vi "Test Copy from Pixmap.vi"(8 "error in (no error)":errorcluster, 11 "Test Case In":refnum<class "Image.lvclass">) -> (0 "error out":errorcluster, 3 "Test Case Out":refnum<class "Image.lvclass">)   [LabVIEW 2020, in "g_ar_toolkit.test.lvlib" / "Image.lvclass"]
uses:
  Image.lvclass
  C:/Program Files (x86)/National Instruments/LabVIEW 2020/vi.lib/Astemes/LUnit/Test Case.lvclass
  <vilib>/Astemes/LUnit/Test Case.lvclass/Test Case.ctl
  g_ar_toolkit.image/CreateEmptyImageARGB.vi
  g_ar_toolkit.image/CopyPixmapToImageIgnoreMaskARGB.vi
  4993e8ee-a06a-463a-9684-69129f64d5ce.vi
  g_ar_toolkit.image/CreateEmptyImageARGB.vi/3321fa97-f432-4e1e-8db9-a0df79aed21b.vi
  g_ar_toolkit.image/CopyPixmapToImageIgnoreMaskARGB.vi/80b1166a-8c06-443b-b271-eb6a715622f7.vi
  <vilib>/Astemes/LUnit/Append Pass Result.vi
  <vilib>/Astemes/LUnit/Append Fail Result.vi
  <vilib>/Astemes/LUnit/Describe Comparison.vi
  <vilib>/Astemes/LUnit/Compare Variants.vi
  g_ar_toolkit.image/FixPixmapColourArraySize.vi
  <vilib>/Astemes/LUnit/Variant to string.vi
  g_ar_toolkit.image/Default8bitColourMap.vi
  <vilib>/Utility/Data Type/Get Type Information.vi
  <vilib>/Utility/LVClass/Get LV Class Name.vi
  g_ar_toolkit.image/ARGBColourToU32.vi
  <vilib>/Utility/error.llb/Error Cluster From Error Code.vi
  Image.lvclass/Image.ctl
  g_ar_toolkit.image/g_ar_toolkit.image.lvlib
panel:
  out "output cluster":T1(array[cluster]) {"data value" format="%.0x"; "24-bit pixmap" format="%.0x"}
  out "Array":picture[](array[picture])
  out "data value":u32[][][](array[numeric]) format="%.0x"
  out "Picture":picture
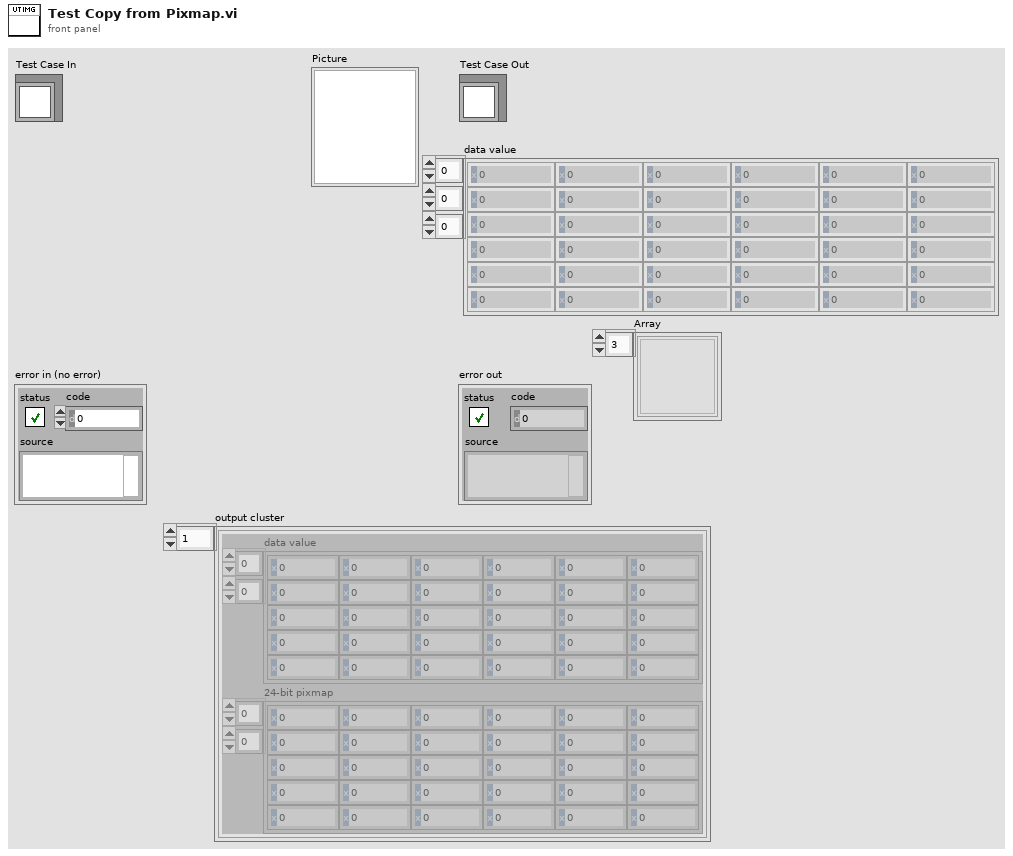
[diagram p1: front panel]
types:
  T1 = cluster{"data value":u32[][], "24-bit pixmap":u32[][]}[]
  T2 = cluster{"left":i16, "top":i16, "right":i16, "bottom":i16}
  T3 = typedef "imagedata.ctl" = cluster{"image type":i32, "image depth":i32, "image":u8[], "mask":u8[], "colors":u32[], "Rectangle":cluster{"left":i16, "top":i16, "right":i16, "bottom":i16}}
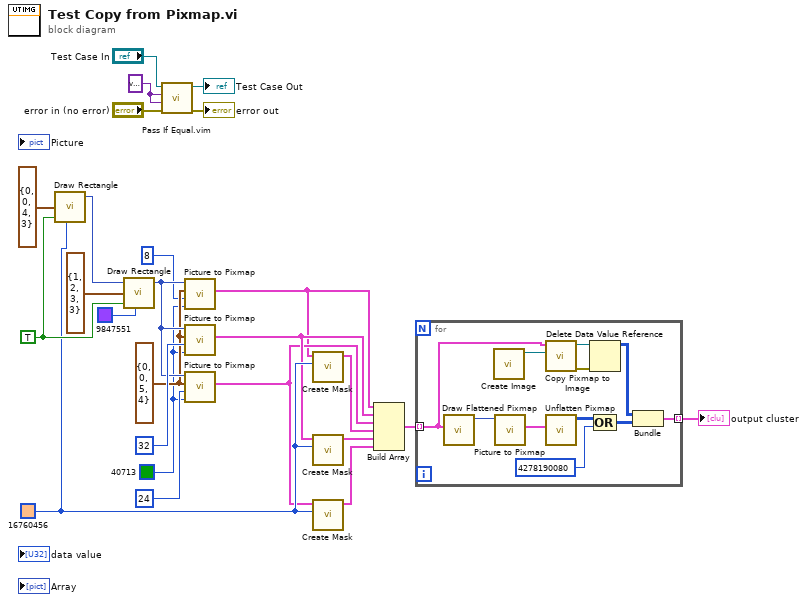
[diagram p0: block diagram]
diagram:
  w15 = TRUE ("fill?(F)")
  w16 = variant ("Expected")
  w12 = T2 {"left"=0, "top"=0, "right"=5, "bottom"=4} ("rect")
  w10 = u32 40713 ("Background Color")
  w9 = u32 16760456 ("color(black)")
  n1 = call <vilib>:"Draw Rectangle.vi"("rect"=T2 {"left"=0, "top"=0, "right"=4, "bottom"=3}, "fill?(F)"=w15, "color(black)"=w9) -> ("new picture"=w21:picture)  [unwired: 6 in]
  n2 = call <vilib>:"Draw Rectangle.vi"("picture"=w21, "rect"=T2 {"left"=1, "top"=2, "right"=3, "bottom"=3}, "fill?(F)"=w15, "color(black)"=u32 9847551) -> ("new picture"=w13:picture)  [unwired: 5 in]
  n3 = call "Pass If Equal.vim"("error in (no error)"="error in (no error)", "Actual"=w16, "Expected"=w16, "LUnit Test Case In"="Test Case In") -> ("error out"=→"error out":errorcluster, "LUnit Test Case Out"=→"Test Case Out":refnum<class "Image.lvclass">)  [unwired: 6 in]
  n4 = call <vilib>:"Picture to Pixmap.vi"("Background Color"=w10, "depth"=8, "rect"=w12, "picture"=w13) -> ("image data"=w1:T3)  [unwired: 6 in, 1 out]
  n5 = call <vilib>:"Picture to Pixmap.vi"("Background Color"=w10, "depth"=32, "rect"=w12, "picture"=w13) -> ("image data"=w8:T3)  [unwired: 6 in, 1 out]
  n6 = call <vilib>:"Picture to Pixmap.vi"("Background Color"=w10, "depth"=24, "rect"=w12, "picture"=w13) -> ("image data"=w2:T3)  [unwired: 6 in, 1 out]
  n7 = call <vilib>:"Create Mask.vi"("Mask Color (Black)"=w9, "image data"=w1) -> ("image data"=w7:T3)  [unwired: 9 in]
  n8 = call <vilib>:"Create Mask.vi"("Mask Color (Black)"=w9, "image data"=w8) -> ("image data"=w6:T3)  [unwired: 9 in]
  n9 = call <vilib>:"Create Mask.vi"("Mask Color (Black)"=w9, "image data"=w2) -> ("image data"=w5:T3)  [unwired: 9 in]
  n10 = Build Array(w1, w8, w2, w7, w6, w5) -> (w4:T3[])
  n11 = for {
    tunnel: w4 -> [w29] mode=indexing
    tunnel: [w30] -> w3 mode=indexing
    n12 = call <vilib>:"Draw Flattened Pixmap.vi"("image data"=w29) -> ("new picture"=w36:picture)  [unwired: 8 in]
    n13 = call-poly "Create Image.vi"() -> ("New ARGB Image"=w32:refnum<data-value>)  [unwired: 10 in, 1 out]
    n14 = call <vilib>:"Picture to Pixmap.vi"("picture"=w36) -> ("image data"=w35:T3)  [unwired: 9 in, 1 out]
    n15 = call-poly "Copy Pixmap to Image.vi"("ARGB Image Destination"=w32, "Pixmap Image Data"=w29) -> ("error out"=w34:errorcluster, "ARGB Image Destination (duplicate)"=w33:refnum<data-value>)  [unwired: 8 in]
    n16 = call <vilib>:"Unflatten Pixmap.vi"("image data"=w35) -> ("24-bit pixmap"=w28:u32[][])  [unwired: 4 in, 6 out]
    n17 = Delete Data Value Reference(data value reference=w33, error in=w34) -> (data value=w31:u32[][])  [unwired: 1 out]
    n18 = Compound Arithmetic op=OR(w28, u32 4278190080) -> (w27:u32[][])
    n19 = Bundle("data value"=w31, w27) -> (w30:cluster{"data value":u32[][], u32[][]})  [unwired: 1 in]
  }
  "output cluster" <- w3
